vi "Connect.vi"(8 "error in (no error)":errorcluster, 9 "timeout":i32=-1, 11 "Network Stream Initiator in":refnum<class "Network Stream Initiator.lvclass">) -> (0 "error out":errorcluster, 3 "Network Stream Initiator out":refnum<class "Network Stream Initiator.lvclass">)   [LabVIEW 2020, in "Network Stream Initiator.lvclass"]
doc: "This method initiates a connection between a Network Stream Initiator/Listener pair."
uses:
  <vilib>/NI/Actors/Network Endpoint Actors/Protocols/Network Stream Strategy/Network Stream Initiator/Network Stream Initiator.lvclass
  C:/Program Files (x86)/National Instruments/LabVIEW 2020/vi.lib/NI/Actors/Network Endpoint Actors/Protocols/Network Stream Strategy/Network Stream/Network Stream.lvclass
  <vilib>/NI/Actors/Network Endpoint Actors/Protocols/Network Stream Strategy/Network Stream/Network Stream.lvclass/Network Stream.ctl
  <vilib>/NI/Actors/Network Endpoint Actors/Protocols/Network Stream Strategy/Network Stream Initiator/Network Stream Initiator.lvclass/Network Stream Initiator.ctl
  <vilib>/NI/Actors/Network Endpoint Actors/Protocols/Network Stream Strategy/Network Stream/Network Stream.lvclass
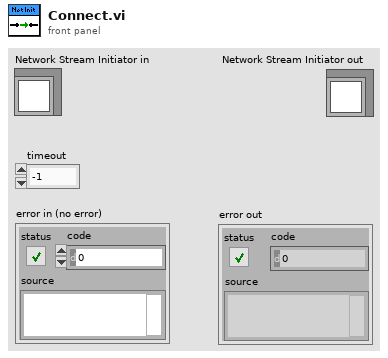
[diagram p1: front panel]
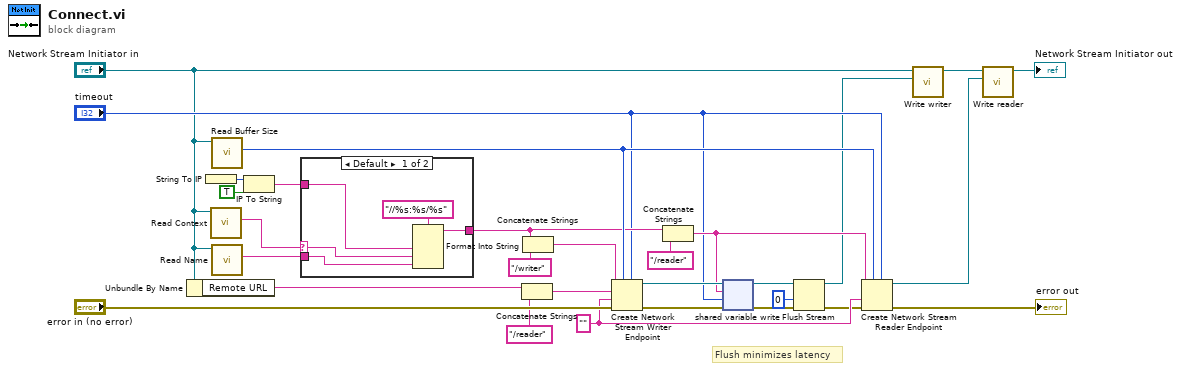
[diagram p0: block diagram]
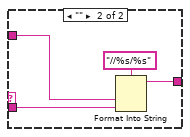
[diagram p2: hidden frame]
diagram:
  w23 = ""
  # "Flush minimizes latency"
  n1 = Unbundle By Name("Network Stream Initiator in") -> ("Remote URL"=w28:string)
  n2 = String To IP() -> (0:w8:u32)  [unwired: 1 in]
  n3 = call <vilib>:"Read Context.vi"("Network Stream in"="Network Stream Initiator in") -> ("Context"=w26:string)  [unwired: 10 in]
  n4 = call <vilib>:"Read Buffer Size.vi"("Network Stream in"="Network Stream Initiator in") -> ("Buffer Size"=w24:i32)  [unwired: 10 in]
  n5 = call <vilib>:"Read Name.vi"("Network Stream in"="Network Stream Initiator in") -> ("Name"=w27:string)  [unwired: 10 in]
  n6 = IP To String(1:TRUE ("dot notation? (F)"), 2:w8) -> (0:w6:string)
  n7 = case shown="Default" w26 {
    selector: w26 -> [w31 _]
    tunnel: [w33 w38] -> w17
    tunnel: w27 -> [w32 w36]
    tunnel: w6 -> [w30 w35]
    frame Default {
      n8 = Format Into String(format string="//%s:%s/%s", w30, w31, w32) -> (resulting string=w33:string)  [unwired: 2 in, 1 out]
    }
    frame "" {
      n9 = Format Into String(format string="//%s/%s", w35, w36) -> (resulting string=w38:string)  [unwired: 2 in, 1 out]
    }
  }
  n10 = Concatenate Strings(w28, "/reader" ("format string")) -> (w21:string)
  n11 = Concatenate Strings(w17, "/writer" ("format string")) -> (w19:string)
  n12 = Create Network Stream Writer Endpoint(5:"timeout", 7:w24, 8:"error in (no error)", 9:w23, 10:w21, 11:w19) -> (0:w16:errorcluster, 3:w15:refnum<k21>)  [unwired: 1 in]
  n13 = Concatenate Strings(w17, "/reader" ("format string")) -> (w14:string)
  n14 = shared-variable-write(w15, w16, w14, "timeout") -> (w2:refnum<k21>, w4:errorcluster)  [unwired: 1 out]
  n15 = Flush Stream(8:w4, 9:0 ("timeout in ms (-1)"), 11:w2) -> (0:w3:errorcluster, 3:w1:refnum<k21>)  [unwired: 1 in, 1 out]
  n16 = Create Network Stream Reader Endpoint(5:"timeout", 7:w24, 8:w3, 9:w23, 11:w14) -> (0:→"error out":errorcluster, 3:w12:refnum<k21>)  [unwired: 2 in]
  n17 = call <vilib>:"Write writer.vi"("writer"=w1, "Network Stream in"="Network Stream Initiator in") -> ("Network Stream out"=w10:refnum<class "Network Stream Initiator.lvclass">)  [unwired: 9 in]
  n18 = call <vilib>:"Write reader.vi"("reader"=w12, "Network Stream in"=w10) -> ("Network Stream out"=→"Network Stream Initiator out":refnum<class "Network Stream Initiator.lvclass">)  [unwired: 9 in]
